vi "2048.vi"() -> ()   [LabVIEW 2020]
panel:
  out "最高分":dbl
  in  "重新开始":bool
  out "得分":dbl
  in  "退出按钮":bool caption="空白按钮"
  out "2048数组":u16[][](array[ring])
  # "2048   v1.0 beta"
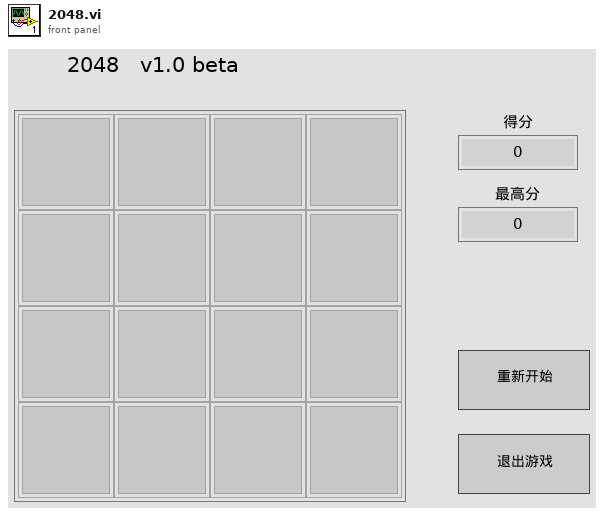
[diagram p1: front panel]
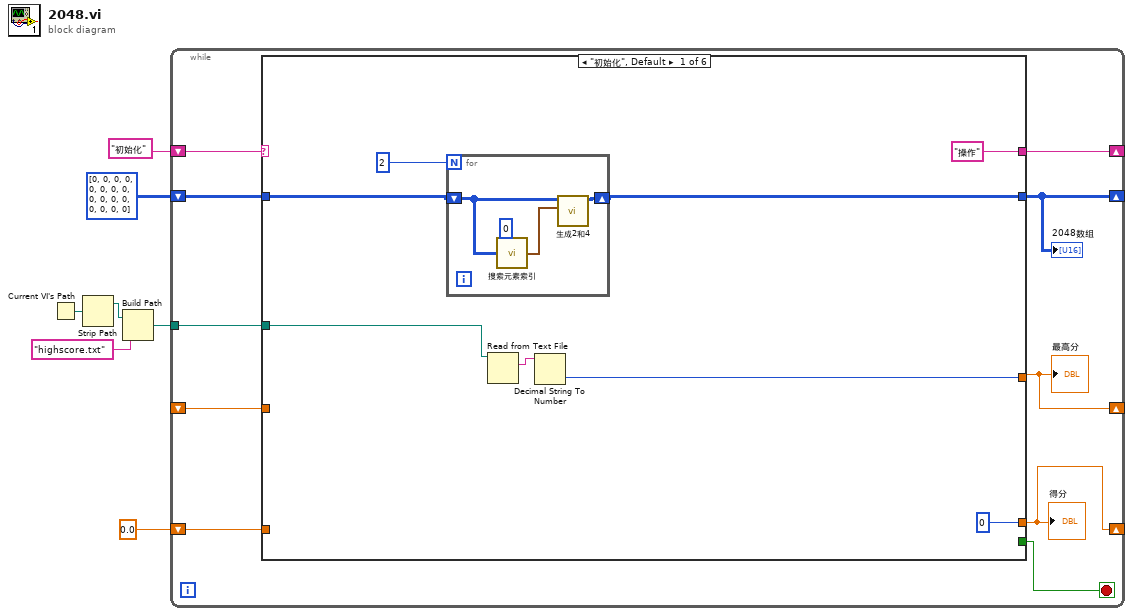
[diagram p0: block diagram]
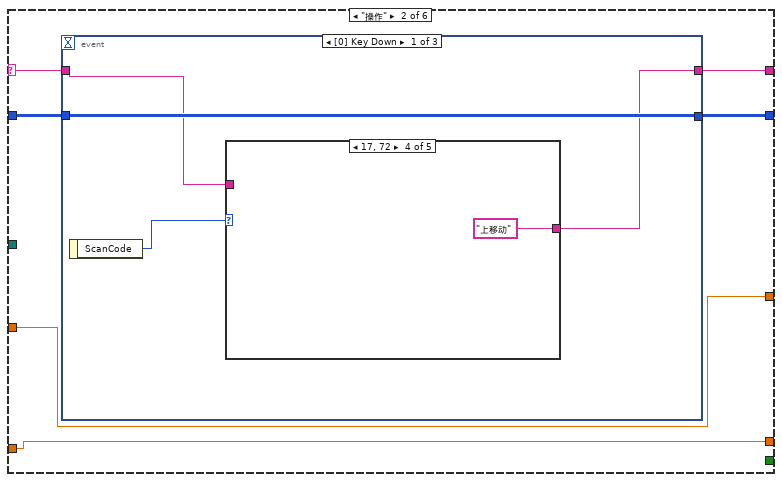
[diagram p2: hidden frame]
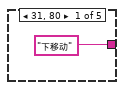
[diagram p3: hidden frame]
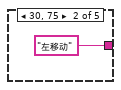
[diagram p4: hidden frame]
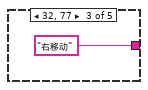
[diagram p5: hidden frame]
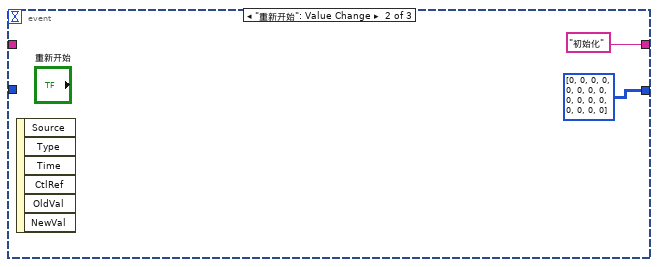
[diagram p7: hidden frame]
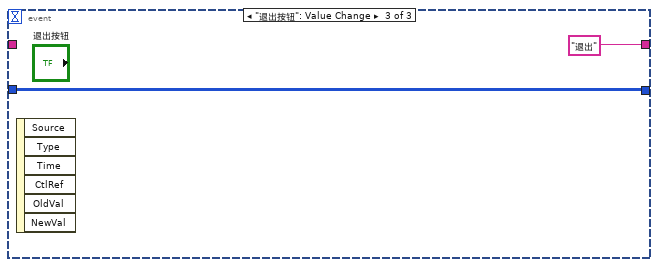
[diagram p8: hidden frame]
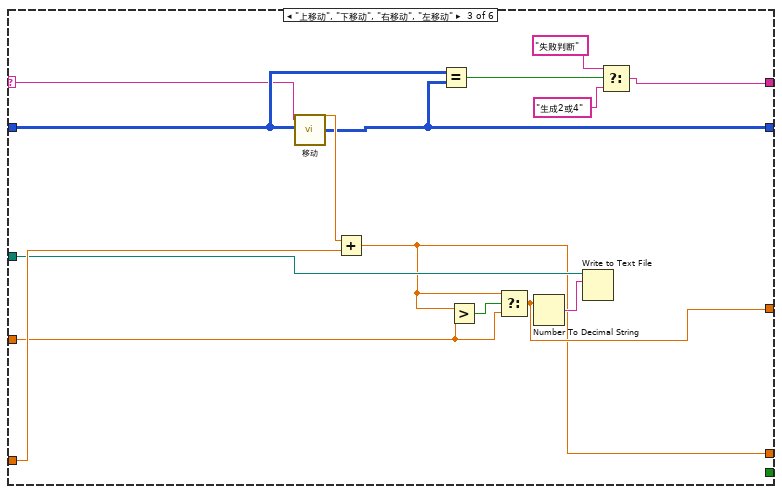
[diagram p9: hidden frame]
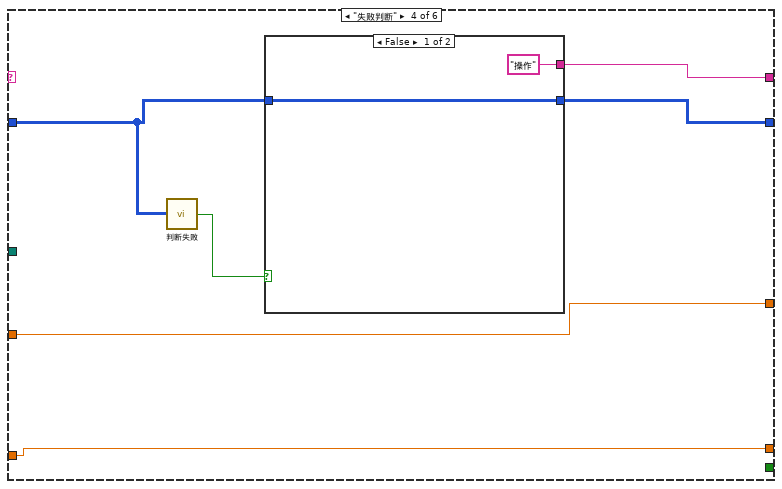
[diagram p10: hidden frame]
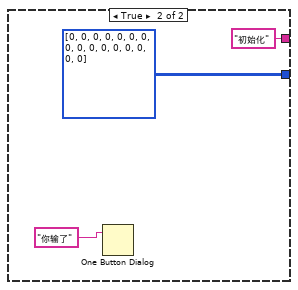
[diagram p11: hidden frame]
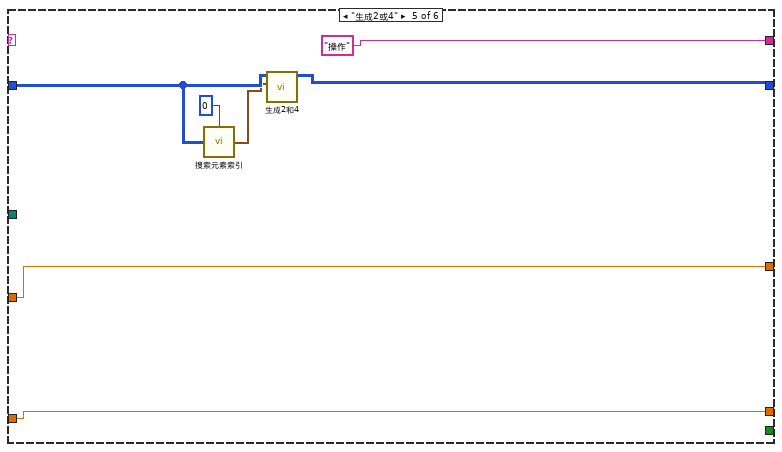
[diagram p12: hidden frame]
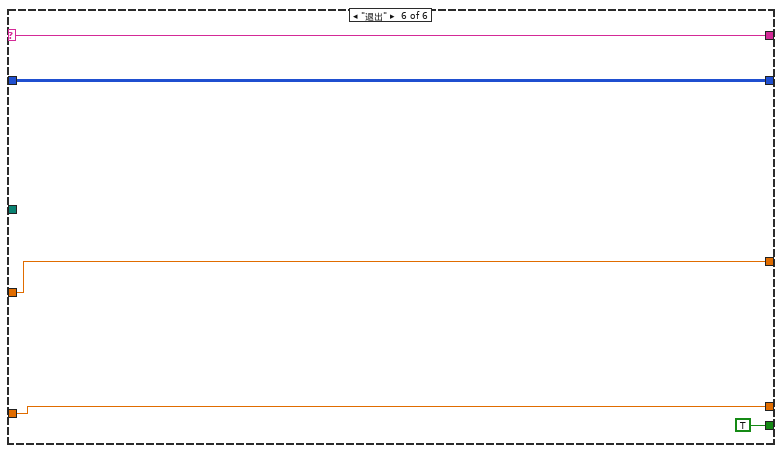
[diagram p13: hidden frame]
diagram:
  n1 = Current VI's Path() -> (path=w4:path)
  n2 = Strip Path(path=w4) -> (stripped path=w3:path)  [unwired: 1 out]
  n3 = Build Path(base path=w3, name or relative path="highscore.txt") -> (appended path=w1:path)
  n4 = while {
    shift-right: [w13] -> _
    shift-left: i32[][] [[0, 0, 0, 0], [0, 0, 0, 0], [0, 0, 0, 0], [0, 0, 0, 0]] -> [w17]
    shift-right: [w15] -> _
    shift-left: "初始化" -> [w16]
    shift-right: [w11] -> _
    shift-left: 0.0 -> [w14]
    tunnel: w1 -> [w10]
    shift-right: [w9] -> _
    shift-left: _ -> [w8]
    stop <- w12 stop-if-true
    n5 = case shown="\"初始化\", Default" w16 {
      selector: w16 -> [_ w32 w58 _ _ w86]
      tunnel: w17 -> [w21 w33 w59 w66 w78 w84]
      tunnel: [w22 w35 w56 w68 w76 w84] -> w13
      tunnel: ["操作" w34 w60 w69 "操作" w86] -> w15
      tunnel: w14 -> [_ w31 w52 w65 w80 w85]
      tunnel: [0 w31 w49 w65 w80 w85] -> w11
      tunnel: [_ _ _ _ _ TRUE] -> w12
      tunnel: w10 -> [w19 _ w50 _ _ _]
      tunnel: [w18 w30 w53 w64 w75 w82] -> w9
      tunnel: w8 -> [_ w30 w51 w64 w75 w82]
      frame "初始化", Default {
        n6 = for {
          N: 2 -> [_]
          shift-right: [w28] -> w22
          shift-left: w21 -> [w26]
          n7 = call "搜索元素索引.vi"("搜索值"=0, "数组"=w26) -> ("索引簇"=w27:cluster{i32, i32}[])  [unwired: 2 in]
          n8 = call "生成2和4.vi"("索引数组"=w27, "2048输入"=w26) -> ("2048输出"=w28:i32[][])  [unwired: 9 in]
        }
        n9 = Read from Text File(file (use dialog)=w19) -> (text=w20:string)  [unwired: 3 in, 3 out]
        n10 = Decimal String To Number(string=w20) -> (number=w18:i32)  [unwired: 2 in, 1 out]
      }
      frame "操作" {
        n11 = event shown="[0] Key Down" {
          selector: _ -> [_ _ _]
          dyn-events: _ -> [_ _ _]
          timeout: _ -> [_ _ _]
          tunnel: [w39 i32[][] [[0, 0, 0, 0], [0, 0, 0, 0], [0, 0, 0, 0], [0, 0, 0, 0]] w48] -> w35
          tunnel: [w37 "初始化" "退出"] -> w34
          tunnel: w33 -> [w39 _ w48]
          tunnel: w32 -> [w36 _ _]
          event Key Down {
            n12 = event-data() -> ("ScanCode"=w38:i16)  [unwired: 1 in]
            n13 = case shown="17, 72" w38 {
              tunnel: ["下移动" "左移动" "右移动" "上移动" w44] -> w37
              tunnel: w36 -> [_ _ _ _ w44]
              frame 31, 80 {
              }
              frame 30, 75 {
              }
              frame 32, 77 {
              }
              frame 17, 72 {
              }
              frame 0, Default {
              }
            }
          }
          event "重新开始": Value Change {
            n14 = event-data() -> ()  [unwired: 1 in, 6 out]
          }
          event "退出按钮": Value Change {
            n15 = event-data() -> ()  [unwired: 1 in, 6 out]
          }
        }
      }
      frame "上移动", "下移动", "右移动", "左移动" {
        n16 = call "移动.vi"("移动前"=w59, "移动方式"=w58) -> ("移动后"=w56:i32[][], "分数"=w57:ext)  [unwired: 1 in]
        n17 = Add(x=w57, y=w52) -> (x+y=w49:ext)
        n18 = Equal?(x=w59, y=w56) -> (x = y?=w63:bool)
        n19 = Greater?(x=w49, y=w51) -> (0:w54:bool)
        n20 = Select(t=w49, s=w54, f=w51) -> (s? t:f=w53:ext)
        n21 = Number To Decimal String(number=w53) -> (decimal integer string=w55:string)  [unwired: 1 in]
        n22 = Write to Text File(file (use dialog)=w50, text=w55) -> ()  [unwired: 2 in, 3 out]
        n23 = Select(t="失败判断", s=w63, f="生成2或4") -> (s? t:f=w60:string)
      }
      frame "失败判断" {
        n24 = call "判断失败.vi"("数组"=w66) -> ("布尔"=w67:bool)
        n25 = case shown="False" w67 {
          tunnel: ["操作" "初始化"] -> w69
          tunnel: [w70 i32[][] [[0, 0, 0, 0], [0, 0, 0, 0], [0, 0, 0, 0], [0, 0, 0, 0]] ("2048")] -> w68
          tunnel: w66 -> [w70 _]
          frame False {
          }
          frame True {
            n26 = One Button Dialog(message="你输了" ("消息")) -> ()  [unwired: 1 in, 1 out]
          }
        }
      }
      frame "生成2或4" {
        n27 = call "搜索元素索引.vi"("搜索值"=0, "数组"=w78) -> ("索引簇"=w77:cluster{i32, i32}[])  [unwired: 2 in]
        n28 = call "生成2和4.vi"("索引数组"=w77, "2048输入"=w78) -> ("2048输出"=w76:i32[][])  [unwired: 9 in]
      }
      frame "退出" {
      }
    }
    "2048数组" <- w13
    "得分" <- w11
    "最高分" <- w9
  }
